vi "Animation time comparator.vi"(8 "Animation":i32, 10 "Velocity in":dbl, 11 "Energy":dbl) -> (0 "Velocity out":dbl, 2 "Energy out":dbl)   [LabVIEW 2020]
doc: "After proton's animation hits edge of windows it needs to begin anew. This SubVI resets values of energy and velocity inside shift registers. \nAnimation - status of animation \nEnergy/Velocity in: if animation has not exceeded they remaing the same\nEnergy/ Velocity out - as above"
uses:
  Global variables.vi
panel:
  # "This SubVi resets energy back to starting, if proton is excessing animation"
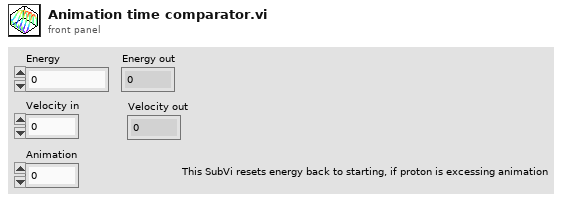
[diagram p1: front panel]
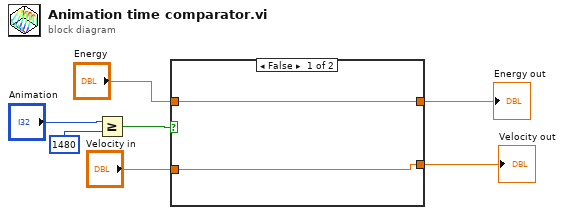
[diagram p0: block diagram]
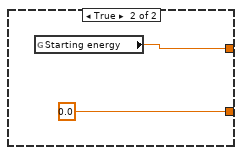
[diagram p2: hidden frame]
diagram:
  n1 = Greater Or Equal?(x="Animation", y=1480) -> (x >= y?=w5:bool)
  n2 = case shown="False" w5 {
    tunnel: [w9 w11] -> w6
    tunnel: "Energy" -> [w9 _]
    tunnel: [w8 0.0] -> w4
    tunnel: "Velocity in" -> [w8 _]
    frame False {
    }
    frame True {
      n3 = global read "Global variables.vi" "Starting energy"() -> (w11:dbl)
    }
  }
  "Energy out" <- w6
  "Velocity out" <- w4
